vi "get_parameter.vi"(0 "HGF_VariantDataObject":refnum<class "HGF_VariantDataObject.lvclass">, 5 "error in (no error)":errorcluster) -> (14 "dup HGF_VariantDataObject":refnum<class "HGF_VariantDataObject.lvclass">, 16 "parameter":variant, 17 "typeDescriptor":string, 19 "error out":errorcluster)   [LabVIEW 2014, in "HGF_BaseClasses.lvlib" / "HGF_VariantDataObject.lvclass"]
doc: "Get Parameter."
uses:
  HGF_VariantDataObject.lvclass
  HGF_VariantDataObject.lvclass/HGF_VariantDataObject.ctl
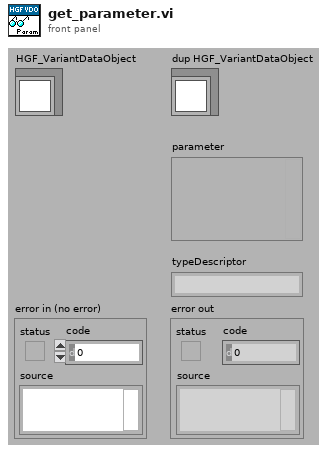
[diagram p1: front panel]
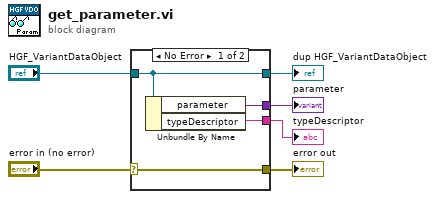
[diagram p0: block diagram]
diagram:
  n1 = case shown="No Error" "error in (no error)" {
    selector: "error in (no error)" -> [w10 w11]
    tunnel: [w10 w11] -> w5
    tunnel: [w9 w12] -> w3
    tunnel: "HGF_VariantDataObject" -> [w9 w12]
    tunnel: [w8 _] -> w2
    tunnel: [w7 _] -> w1
    frame No Error {
      n2 = Unbundle By Name(w9) -> ("parameter"=w8:variant, "typeDescriptor"=w7:string)
    }
    frame Error {
    }
  }
  "error out" <- w5
  "dup HGF_VariantDataObject" <- w3
  "parameter" <- w2
  "typeDescriptor" <- w1
